vi "Omniax_mDrive_GNDRead.vi"() -> ()   [LabVIEW 2015]
uses:
  Omniax_mDrive_GNDGlobal.vi
panel:
  out "sample NC":bool
  in  "stop":bool
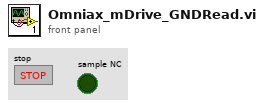
[diagram p1: front panel]
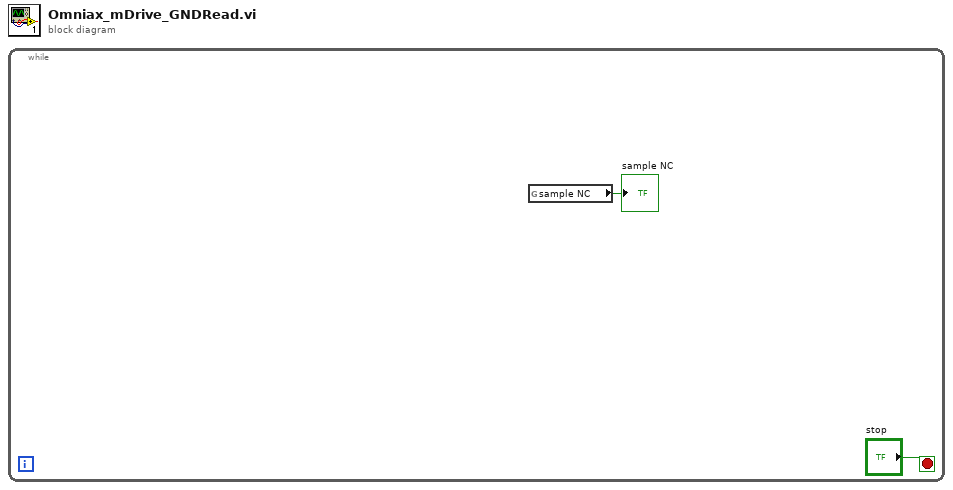
[diagram p0: block diagram]
diagram:
  n1 = while {
    stop <- "stop" stop-if-true
    n2 = global read "Omniax_mDrive_GNDGlobal.vi" "sample NC"() -> (→"sample NC":bool)
  }
